vi "XY Graph Delete Plot Event.vi"(8 "Error In":errorcluster, 9 "Mouse Click Coordinates":T1, 11 "XYGraph Ref":T2) -> (0 "Error Out":errorcluster, 1 "Message":string, 2 "Plot Name":string, 3 "Deleted Plot Index":i32, 5 "Graph Caption":string)   [LabVIEW 2019, in "XY Graph Add-Ons.lvlib"]
uses:
  XY Graph Add-Ons.lvlib
  XY Graph Refnum.ctl
  <vilib>/Utility/miscctls.llb/LVPoint32TypeDef.ctl
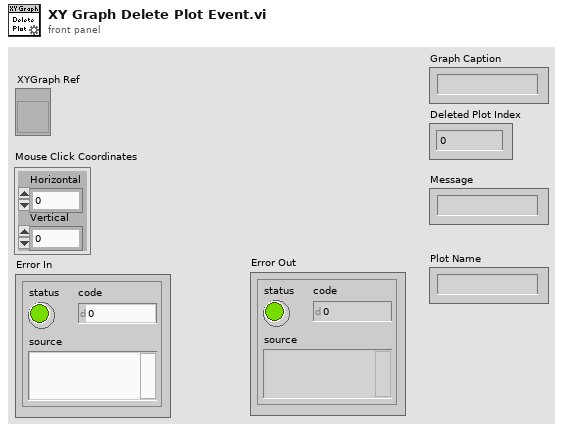
[diagram p1: front panel]
types:
  T1 = typedef "LVPoint32TypeDef.ctl" = cluster{"Horizontal":i32, "Vertical":i32}
  T2 = typedef "XY Graph Add-Ons.lvlib/XY Graph Refnum.ctl" = refnum<vi>
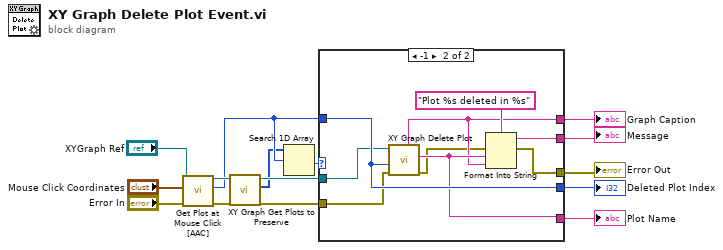
[diagram p0: block diagram]
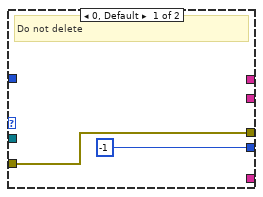
[diagram p2: hidden frame]
diagram:
  n1 = call "Get Plot at Mouse Click [AAC].vi"("error in (no error)"="Error In", "Mouse Click Coordinates"="Mouse Click Coordinates", "XYGraph Ref"="XYGraph Ref") -> ("error out"=w6:errorcluster, "Plot at Coordinates"=w2:i32, "XYGraph Ref"=w4:T2)  [unwired: 2 in, 4 out]
  n2 = call "XY Graph Get Plots to Preserve.vi"("Error In"=w6, "XYGraph in"=w4) -> ("Error Out"=w5:errorcluster, "Preserved Plots"=w1:i32[], "XYGraph out"=w3:T2)  [unwired: 6 in, 1 out]
  n3 = Search 1D Array(1D array=w1, element=w2) -> (index of element=w12:i32)  [unwired: 1 in]
  n4 = case shown="-1" w12 {
    tunnel: w3 -> [_ w25]
    tunnel: w5 -> [w17 w24]
    tunnel: [w17 w19] -> w11
    tunnel: w2 -> [_ w26]
    tunnel: [-1 ("Plot at Coordinates") w26] -> w10
    tunnel: [_ w21] -> w9
    tunnel: [_ w22] -> w8
    tunnel: [_ w18] -> w7
    frame 0, Default {
      # "Do not delete"
    }
    frame -1 {
      n5 = call "XY Graph Delete Plot.vi"("Error In"=w24, "Plot Index"=w26, "XYGraph Ref"=w25) -> ("Error Out"=w20:errorcluster, "Plot Name"=w22:string, "Graph Caption (or Label)"=w21:string)  [unwired: 5 in, 1 out]
      n6 = Format Into String(format string="Plot %s deleted in %s", error in=w20, w22, w21) -> (resulting string=w18:string, error out=w19:errorcluster)  [unwired: 1 in]
    }
  }
  "Error Out" <- w11
  "Deleted Plot Index" <- w10
  "Graph Caption" <- w9
  "Plot Name" <- w8
  "Message" <- w7
